vi "GetGrabbedWindow.vi"(8 "No Error":errorcluster) -> (0 "Error Out":errorcluster, 3 "Window [SDL_Window *]":i64 format="%.0x")   [LabVIEW 2026, in "SDL3.lvlib" / "Video.lvlib"]
doc: "<B>Summary</B>\nGet the window that currently has an input grab enabled."
uses:
  Video.lvlib
  Lib/SDL3.dll
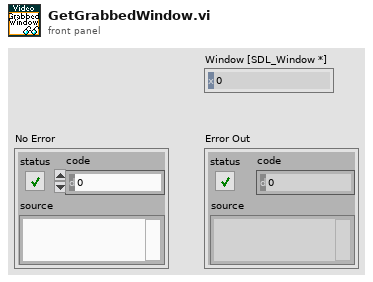
[diagram p1: front panel]
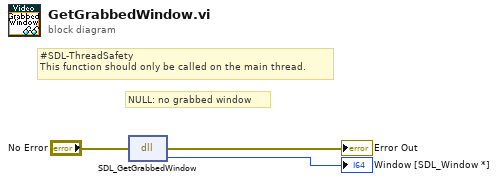
[diagram p0: block diagram]
diagram:
  # "#SDL-ThreadSafety\nThis function should only be called on the main thread."
  # "NULL: no grabbed window"
  n1 = dll-call lib="C:/Users/saukko/Dev/LV-SDL3/Sources/SDL3/Lib/SDL3.*" fn="SDL_GetGrabbedWindow"(error in="No Error") -> (error out=→"Error Out":errorcluster, "return type"=→"Window [SDL_Window *]":i64)  [unwired: 2 in, 1 out]
